vi "strobe.vi"() -> ()   [LabVIEW 2019]
uses:
  <vilib>/DAQmx/write.llb/DAQmx Write (Counter 1D Ticks 1Chan NSamp).vi
  <vilib>/DAQmx/create/channels.llb/DAQmx Create Channel (CO-Pulse Generation-Ticks).vi
  <vilib>/DAQmx/configure/timing.llb/DAQmx Timing (Implicit).vi
  <vilib>/DAQmx/miscellaneous.llb/DAQmx Fill In Error Info.vi
  <resource>/objmgr/daqmx.rc
panel:
  out "SampTimingType":i32(ring)=10388 items=["Sample Clock"=10388, "Burst Handshake"=12548, "Handshake"=10389, "Implicit"=10451, "On Demand"=10390, "Change Detection"=12504, "Pipelined Sample Clock"=14668]
  out "SampClk.Src":tag
  out "output tick cluster":cluster{"high ticks":i32, "low ticks":i32}
  out "TotalSampPerChanGenerated":dbl
  out "Numeric 2":i32
  out "Numeric":i32
  in  "stop":bool
  in  "base scalar":dbl=1000.0 format="%#_13g"
  out "32bit integer":i32
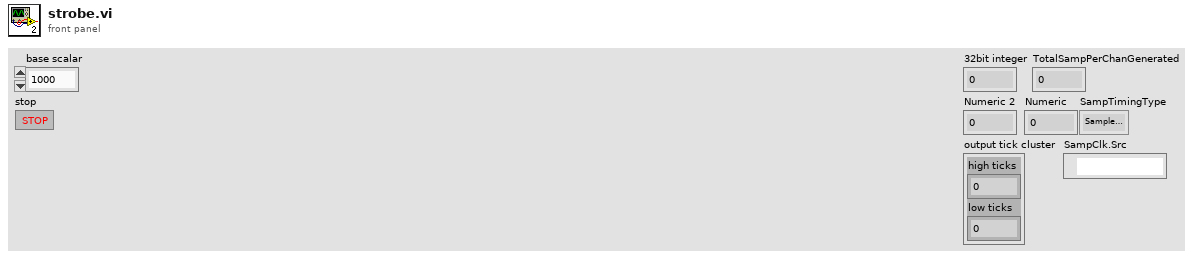
[diagram p1: front panel]
types:
  T1 = cluster{"inner index":i32, "outer index":i32, "array":i32[], "value":bool, "count":i32}
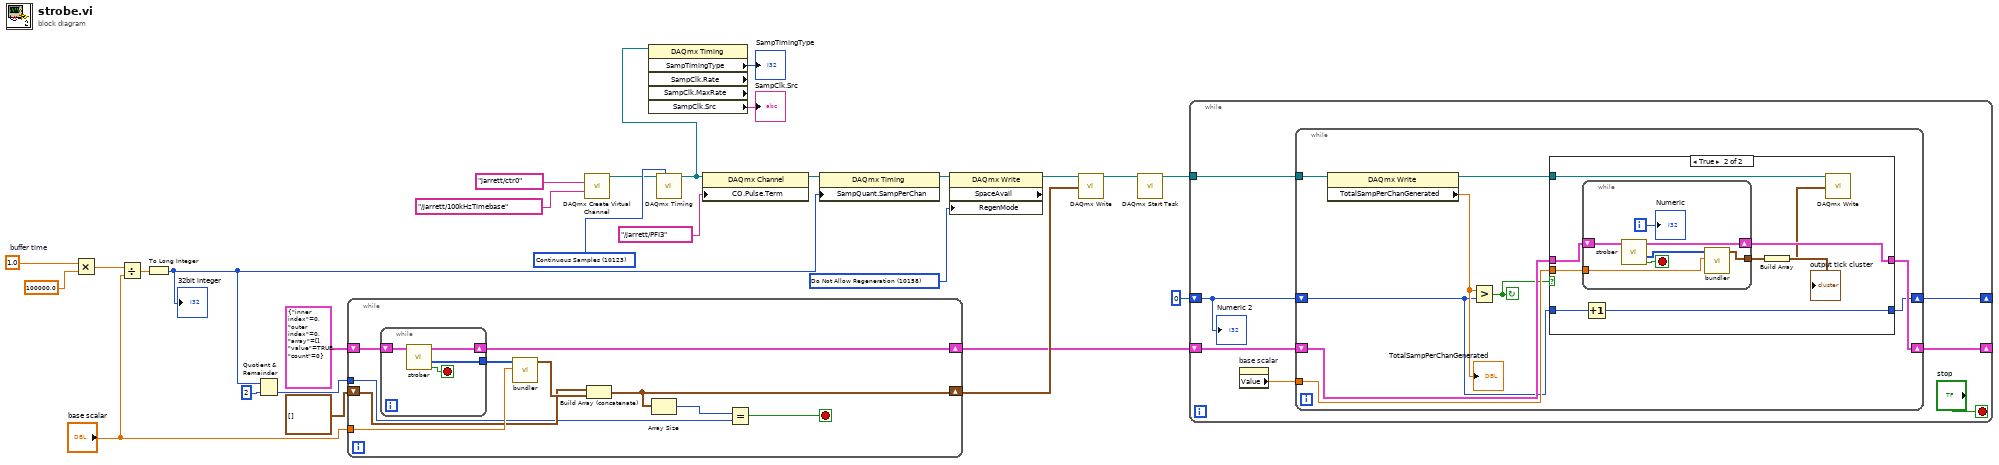
[diagram p0: block diagram]
diagram:
  w9 = 10158 items=["Allow Regeneration"=10097, "Do Not Allow Regeneration"=10158] ("RegenMode")
  w23 = 1.0  # buffer time
  w27 = 10123 items=["Finite Samples"=10178, "Continuous Samples"=10123, "Hardware Timed Single Point"=12522] ("sample mode")
  n1 = Multiply(x=w23, y=100000.0) -> (x*y=w22:dbl)
  n2 = Divide(x=w22, y="base scalar") -> (x/y=w21:dbl)
  n3 = To Long Integer(number=w21) -> (32bit integer=w19:i32)
  "32bit integer" <- w19
  n4 = Quotient & Remainder(x=w19, y=2) -> (floor(x/y)=w13:i32)  [unwired: 1 out]
  n5 = while {
    shift-right: [w36] -> w10
    shift-left: T1 {"inner index"=0, "outer index"=0, "array"=[], "value"=TRUE, "count"=0} ("input reference") -> [w37]
    tunnel: "base scalar" -> [w34]
    shift-right: [w29] -> w12
    shift-left: cluster{"high ticks":i32, "low ticks":i32}[] [] -> [w32]
    tunnel: w13 -> [w28]
    stop <- w30 stop-if-true
    n6 = while {
      shift-right: [w39] -> w36
      shift-left: w37 -> [w41]
      tunnel: [w38] -> w35
      stop <- w40 stop-if-true
      n7 = call "strober.vi"("input reference"=w41) -> ("new data"=w40:bool, "output ticks"=w38:i32[], "output reference"=w39:T1)  [unwired: 8 in]
    }
    n8 = call "bundler.vi"("scalar"=w34, "input ticks"=w35) -> ("output tick cluster"=w33:cluster{"high ticks":i32, "low ticks":i32})  [unwired: 9 in]
    n9 = Build Array (concatenate)(w32, w33) -> (w29:cluster{"high ticks":i32, "low ticks":i32}[])
    n10 = Array Size(array=w29) -> (size(s)=w31:i32)
    n11 = Equal?(x=w31, y=w28) -> (x = y?=w30:bool)
  }
  n12 = call-poly <vilib>:"DAQmx Create Virtual Channel.vi"("counter"=tag "jarrett/ctr0", "source of ticks"=tag "/jarrett/100kHzTimebase") -> ("task out"=w2:refnum<k21>)  [unwired: 12 in, 1 out]
  n13 = call-poly <vilib>:"DAQmx Timing.vi"("task/channels in"=w2, "sample mode"=w27) -> ("task out"=w1:refnum<k21>)  [unwired: 12 in, 1 out]
  n14 = property class="DAQmx Timing" props=["SampTimingType", "SampClk.Rate", "SampClk.MaxRate", "SampClk.Src"](reference=w1) -> ("SampTimingType"=→"SampTimingType":i32, "SampClk.Src"=→"SampClk.Src":tag)  [unwired: 1 in, 4 out]
  n15 = property class="DAQmx Channel"(reference=w1, "CO.Pulse.Term"=tag "/jarrett/PFI3") -> (reference out=w18:refnum<k21>)  [unwired: 1 in, 1 out]
  n16 = property class="DAQmx Timing"(reference=w18, "SampQuant.SampPerChan"=w19) -> (reference out=w8:refnum<k21>)  [unwired: 1 in, 1 out]
  n17 = property class="DAQmx Write" props=["SpaceAvail", "RegenMode"](reference=w8, "RegenMode"=w9) -> (reference out=w7:refnum<k21>)  [unwired: 1 in, 2 out]
  n18 = call-poly <vilib>:"DAQmx Write.vi"("task/channels in"=w7, "data"=w12) -> ("task out"=w6:refnum<k21>)  [unwired: 11 in, 2 out]
  n19 = call <vilib>:"DAQmx Start Task.vi"("task/channels in"=w6) -> ("task out"=w11:refnum<k21>)  [unwired: 13 in, 1 out]
  n20 = while {
    tunnel: w11 -> [w47]
    shift-right: [w45] -> _
    shift-left: w10 -> [w46]
    shift-right: [w42] -> _
    shift-left: 0 -> [w43]
    stop <- "stop" stop-if-true
    n21 = property on="base scalar" class="DigNum (strict)"() -> ("Value"=w44:dbl)  [unwired: 2 in, 2 out]
    n22 = while {
      tunnel: w47 -> [w57]
      shift-right: [w55] -> w45
      shift-left: w46 -> [w56]
      tunnel: w44 -> [w54]
      shift-right: [w49] -> w42
      shift-left: w43 -> [w50]
      stop <- w51 continue-if-true
      n23 = property class="DAQmx Write"(reference=w57) -> (reference out=w53:refnum<k21>, "TotalSampPerChanGenerated"=w52:dbl)  [unwired: 1 in, 1 out]
      "TotalSampPerChanGenerated" <- w52
      n24 = Greater?(x=w52, y=w50) -> (0:w51:bool)
      n25 = case shown="True" w51 {
        tunnel: w56 -> [w59 w67]
        tunnel: [w59 w66] -> w55
        tunnel: w54 -> [_ w65]
        tunnel: w53 -> [_ w64]
        tunnel: w50 -> [w58 w61]
        tunnel: [w58 w60] -> w49
        frame False {
        }
        frame True {
          n26 = while {
            shift-right: [w72] -> w66
            shift-left: w67 -> [w74]
            tunnel: w65 -> [w70]
            tunnel: [w69] -> w63
            i -> [w68]
            stop <- w73 stop-if-true
            n27 = call "strober.vi"("input reference"=w74) -> ("new data"=w73:bool, "output ticks"=w71:i32[], "output reference"=w72:T1)  [unwired: 8 in]
            n28 = call "bundler.vi"("scalar"=w70, "input ticks"=w71) -> ("output tick cluster"=w69:cluster{"high ticks":i32, "low ticks":i32})  [unwired: 9 in]
            "Numeric" <- w68
          }
          "output tick cluster" <- w63
          n29 = Increment(x=w61) -> (x+1=w60:i32)
          n30 = Build Array(w63) -> (w62:cluster{"high ticks":i32, "low ticks":i32}[])
          n31 = call-poly <vilib>:"DAQmx Write.vi"("task/channels in"=w64, "data"=w62) -> ()  [unwired: 11 in, 3 out]
        }
      }
    }
    "Numeric 2" <- w43
  }
